vi "PUB-SUB.vi"() -> ()   [LabVIEW 2018]
uses:
  RxTx/CM_RxTx.lvclass
  socket PUB/socket PUB.lvclass
  C:/Users/Denis/Desktop/communication-manager/communication-manager/Socket/Socket.lvclass
  socket SUB/socket SUB.lvclass
  Socket/Socket.lvclass
  <vilib>/addons/zeromq/zmq_context.lvclass
panel:
  out "error out 3":errorcluster
  in  "Queue RX 2":refnum<class "CM_RxTx.lvclass">
  out "Received message":string
  in  "socket SUB.lvclass":refnum<class "socket SUB.lvclass">
  in  "socket PUB.lvclass":refnum<class "socket PUB.lvclass">
  in  "message":string
  in  "send":bool
  out "error out 2":errorcluster
  in  "Queue RX":refnum<class "CM_RxTx.lvclass">
  in  "stop":bool
  # "PUB endpoint"
  # "SUB endpoint"
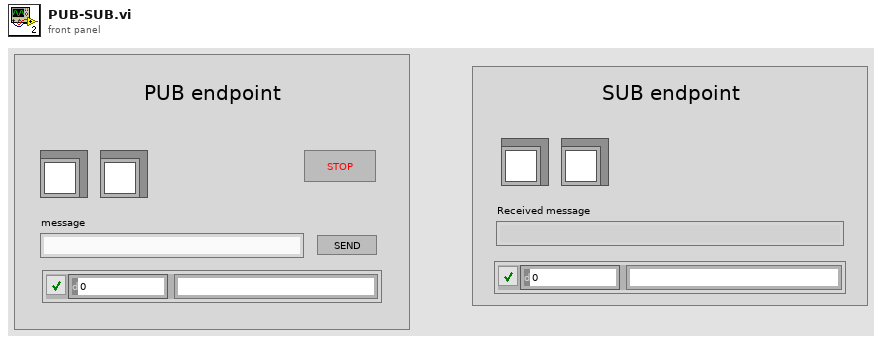
[diagram p1: front panel]
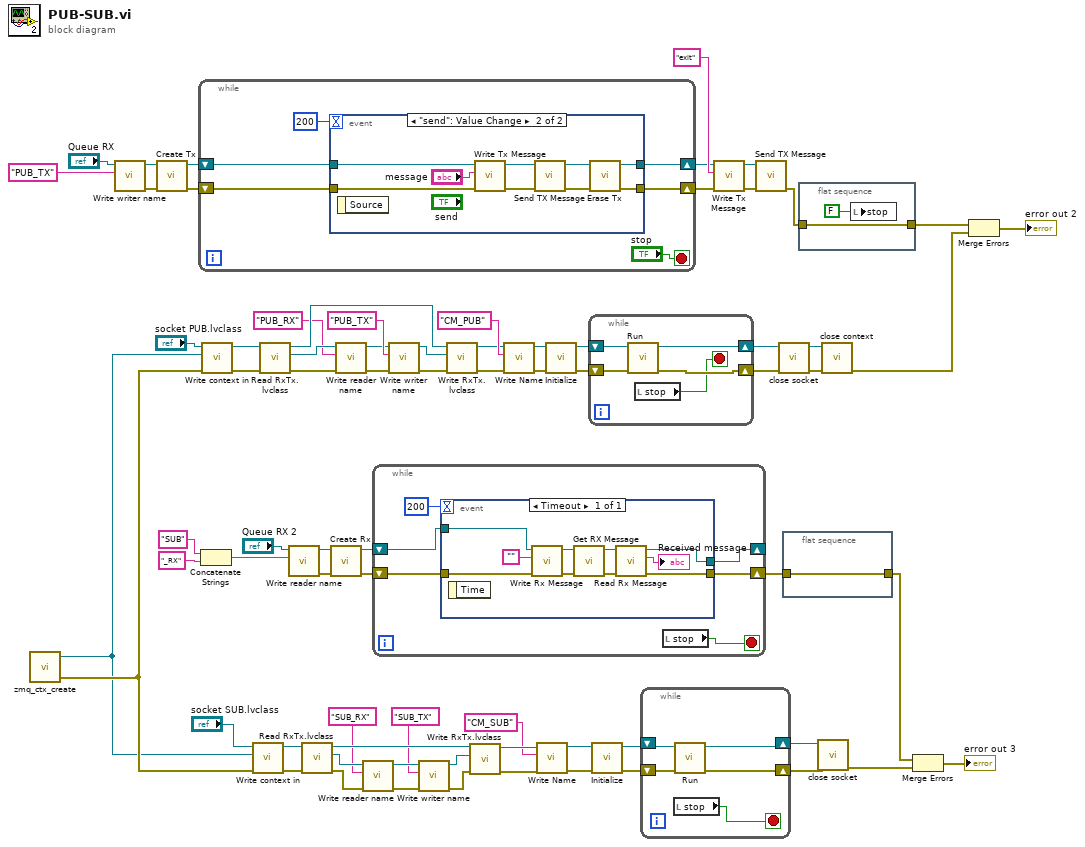
[diagram p0: block diagram]
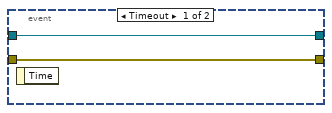
[diagram p2: hidden frame]
diagram:
  n1 = call <vilib>:"zmq_ctx_create.vi"() -> ("error out"=w18:errorcluster, "context out"=w17:refnum<class "zmq_context.lvclass">)  [unwired: 4 in]
  n2 = call-dynamic "Write writer name.vi"("Tx name"="PUB_TX", "RxTx in"="Queue RX") -> ("error out"=w70:errorcluster, "RxTx out"=w71:refnum<class "CM_RxTx.lvclass">)  [unwired: 8 in]
  n3 = call "Create Tx.vi"("error in (no error)"=w70, "RxTx in"=w71) -> ("error out"=w69:errorcluster, "RxTx out"=w73:refnum<class "CM_RxTx.lvclass">)  [unwired: 8 in]
  n4 = while {
    shift-right: [w76] -> w42
    shift-left: w73 -> [w78]
    shift-right: [w75] -> w39
    shift-left: w69 -> [w77]
    stop <- "stop" stop-if-true
    n5 = event shown="[1] \"send\": Value Change" {
      selector: _ -> [_ _]
      dyn-events: _ -> [_ _]
      timeout: 200 -> [_ _]
      tunnel: [w81 w87] -> w76
      tunnel: [w80 w86] -> w75
      tunnel: w78 -> [w81 w83]
      tunnel: w77 -> [w80 w82]
      event Timeout {
        n6 = event-data() -> ()  [unwired: 1 in, 1 out]
      }
      event "send": Value Change {
        n7 = event-data() -> ()  [unwired: 1 in, 1 out]
        n8 = call "Write Tx Message.vi"("error in (no error)"=w82, "Tx Message"="message", "RxTx in"=w83) -> ("error out"=w84:errorcluster, "RxTx out"=w89:refnum<class "CM_RxTx.lvclass">)  [unwired: 7 in]
        n9 = call "Send TX Message.vi"("error in (no error)"=w84, "RxTx in"=w89) -> ("error out"=w85:errorcluster, "RxTx out"=w88:refnum<class "CM_RxTx.lvclass">)  [unwired: 8 in]
        n10 = call "Erase Tx.vi"("error in (no error)"=w85, "RxTx in"=w88) -> ("error out"=w86:errorcluster, "RxTx out"=w87:refnum<class "CM_RxTx.lvclass">)  [unwired: 8 in]
      }
    }
  }
  n11 = Concatenate Strings("SUB" ("string"), "_RX" ("string")) -> (w7:string)
  n12 = call-dynamic "Write context in.vi"("error in (no error)"=w18, "zeromq.lvlib:ZeroMQ Context"=w17, "Socket in"="socket PUB.lvclass") -> ("error out"=w47:errorcluster, "Socket out"=w46:refnum<class "socket PUB.lvclass">)  [unwired: 7 in]
  n13 = call-dynamic "Write context in.vi"("error in (no error)"=w18, "zeromq.lvlib:ZeroMQ Context"=w17, "Socket in"="socket SUB.lvclass") -> ("error out"=w22:errorcluster, "Socket out"=w23:refnum<class "socket SUB.lvclass">)  [unwired: 7 in]
  n14 = call-dynamic "Read RxTx.lvclass.vi"("error in (no error)"=w47, "Socket in"=w46) -> ("error out"=w60:errorcluster, "RxTx.lvclass"=w64:refnum<class "CM_RxTx.lvclass">, "Socket out"=w61:refnum<class "socket PUB.lvclass">)  [unwired: 7 in]
  n15 = call-dynamic "Write reader name.vi"("RX name"=w7, "RxTx in"="Queue RX 2") -> ("error out"=w9:errorcluster, "RxTx out"=w10:refnum<class "CM_RxTx.lvclass">)  [unwired: 8 in]
  n16 = call-dynamic "Read RxTx.lvclass.vi"("error in (no error)"=w22, "Socket in"=w23) -> ("error out"=w30:errorcluster, "RxTx.lvclass"=w26:refnum<class "CM_RxTx.lvclass">, "Socket out"=w29:refnum<class "socket SUB.lvclass">)  [unwired: 7 in]
  n17 = call "Create Rx.vi"("error in (no error)"=w9, "RxTx in"=w10) -> ("error out"=w8:errorcluster, "RxTx out"=w11:refnum<class "CM_RxTx.lvclass">)  [unwired: 8 in]
  n18 = call-dynamic "Write reader name.vi"("error in (no error)"=w60, "RX name"="PUB_RX" ("reader name"), "RxTx in"=w64) -> ("error out"=w59:errorcluster, "RxTx out"=w63:refnum<class "CM_RxTx.lvclass">)  [unwired: 7 in]
  n19 = call-dynamic "Write reader name.vi"("error in (no error)"=w30, "RX name"="SUB_RX" ("reader name"), "RxTx in"=w26) -> ("error out"=w31:errorcluster, "RxTx out"=w27:refnum<class "CM_RxTx.lvclass">)  [unwired: 7 in]
  n20 = while {
    shift-right: [w94] -> _
    shift-left: w11 -> [w95]
    shift-right: [w92] -> w4
    shift-left: w8 -> [w93]
    stop <- w91 stop-if-true
    n21 = event shown="[0] Timeout" {
      selector: _ -> [_]
      dyn-events: _ -> [_]
      timeout: 200 -> [_]
      tunnel: w95 -> [w103]
      tunnel: [w101] -> w94
      tunnel: w93 -> [w98]
      tunnel: [w97] -> w92
      event Timeout {
        n22 = event-data() -> ()  [unwired: 1 in, 1 out]
        n23 = call "Write Rx Message.vi"("error in (no error)"=w98, "Rx Message"="", "RxTx in"=w103) -> ("error out"=w100:errorcluster, "RxTx out"=w102:refnum<class "CM_RxTx.lvclass">)  [unwired: 7 in]
        n24 = call "Get RX Message.vi"("error in (no error)"=w100, "RxTx in"=w102) -> ("error out"=w104:errorcluster, "RxTx out"=w106:refnum<class "CM_RxTx.lvclass">)  [unwired: 7 in, 1 out]
        n25 = call "Read Rx Message.vi"("error in (no error)"=w104, "RxTx in"=w106) -> ("error out"=w97:errorcluster, "Rx Message"=→"Received message":string, "RxTx out"=w101:refnum<class "CM_RxTx.lvclass">)  [unwired: 7 in]
      }
    }
    n26 = local read "stop"() -> (w91:bool)
  }
  n27 = call-dynamic "Write writer name.vi"("error in (no error)"=w59, "Tx name"="PUB_TX" ("writer name"), "RxTx in"=w63) -> ("error out"=w58:errorcluster, "RxTx out"=w62:refnum<class "CM_RxTx.lvclass">)  [unwired: 7 in]
  n28 = call-dynamic "Write writer name.vi"("error in (no error)"=w31, "Tx name"="SUB_TX" ("writer name"), "RxTx in"=w27) -> ("error out"=w32:errorcluster, "RxTx out"=w28:refnum<class "CM_RxTx.lvclass">)  [unwired: 7 in]
  n29 = call-dynamic "Write RxTx.lvclass.vi"("error in (no error)"=w58, "RxTx.lvclass"=w62, "Socket in"=w61) -> ("error out"=w48:errorcluster, "Socket out"=w49:refnum<class "socket PUB.lvclass">)  [unwired: 7 in]
  n30 = call-dynamic "Write RxTx.lvclass.vi"("error in (no error)"=w32, "RxTx.lvclass"=w28, "Socket in"=w29) -> ("error out"=w35:errorcluster, "Socket out"=w34:refnum<class "socket SUB.lvclass">)  [unwired: 7 in]
  n31 = call-dynamic "Write Name.vi"("error in (no error)"=w48, "Name"="CM_PUB", "Socket in"=w49) -> ("error out"=w56:errorcluster, "Socket out"=w57:refnum<class "socket PUB.lvclass">)  [unwired: 7 in]
  n32 = call-dynamic "Write Name.vi"("error in (no error)"=w35, "Name"="CM_SUB", "Socket in"=w34) -> ("error out"=w19:errorcluster, "Socket out"=w20:refnum<class "socket SUB.lvclass">)  [unwired: 7 in]
  n33 = call-dynamic "Initialize.vi"("error in (no error)"=w56, "socket PUB in"=w57) -> ("error out"=w53:errorcluster, "socket PUB out"=w55:refnum<class "socket PUB.lvclass">)  [unwired: 8 in]
  n34 = while {
    shift-right: [w109] -> w54
    shift-left: w55 -> [w111]
    shift-right: [w108] -> w52
    shift-left: w53 -> [w110]
    stop <- w107 stop-if-true
    n35 = call-dynamic "Run.vi"("error in (no error)"=w110, "socket PUB in"=w111) -> ("error out"=w108:errorcluster, "socket PUB out"=w109:refnum<class "socket PUB.lvclass">)  [unwired: 8 in]
    n36 = local read "stop"() -> (w107:bool)
  }
  n37 = call-dynamic "Initialize.vi"("error in (no error)"=w19, "socket SUB in"=w20) -> ("error out"=w15:errorcluster, "socket SUB out"=w16:refnum<class "socket SUB.lvclass">)  [unwired: 8 in]
  n38 = while {
    shift-right: [w114] -> w13
    shift-left: w16 -> [w116]
    shift-right: [w113] -> w14
    shift-left: w15 -> [w115]
    stop <- w112 stop-if-true
    n39 = local read "stop"() -> (w112:bool)
    n40 = call-dynamic "Run.vi"("error in (no error)"=w115, "socket SUB in"=w116) -> ("error out"=w113:errorcluster, "socket SUB out"=w114:refnum<class "socket SUB.lvclass">)  [unwired: 8 in]
  }
  n41 = call "Write Tx Message.vi"("error in (no error)"=w39, "Tx Message"="exit" ("Publication 2"), "RxTx in"=w42) -> ("error out"=w40:errorcluster, "RxTx out"=w43:refnum<class "CM_RxTx.lvclass">)  [unwired: 7 in]
  n42 = call "Send TX Message.vi"("error in (no error)"=w40, "RxTx in"=w43) -> ("error out"=w41:errorcluster)  [unwired: 8 in, 1 out]
  n43 = call "close socket.vi"("error in (no error)"=w52, "Socket in"=w54) -> ("error out"=w67:errorcluster, "Socket out"=w66:refnum<class "socket PUB.lvclass">)  [unwired: 8 in]
  n44 = flat-sequence {
    tunnel: w4 -> [w117]
    tunnel: [w117] -> w3
    frame #0 {
    }
  }
  n45 = flat-sequence {
    tunnel: w41 -> [w119]
    tunnel: [w119] -> w38
    frame #0 {
      n46 = local write "stop"(FALSE ("stop")) -> ()
    }
  }
  n47 = call "close socket.vi"("error in (no error)"=w14, "Socket in"=w13) -> ("error out"=w2:errorcluster)  [unwired: 8 in, 1 out]
  n48 = call-dynamic "close context.vi"("error in (no error)"=w67, "Socket in"=w66) -> ("error out"=w36:errorcluster)  [unwired: 8 in, 1 out]
  n49 = Merge Errors(w3, w2) -> (→"error out 3":errorcluster)
  n50 = Merge Errors(w38, w36) -> (→"error out 2":errorcluster)
